vi "Emphasize Color.vi"(2 "error in 2 (no error)":errorcluster, 3 "Color":i8, 4 "Image Dst":T1, 5 "Image Src":T1) -> (0 "error out":errorcluster, 1 "Image Out":T1)   [LabVIEW 2009, in "ImageProcessing.lvlib"]
doc: "Output is a grayscaled image calculated as\n (255*X)/(R+G+B) \nwhere X is R, G or B depending on what number is showsen in color (0 = R, 1 = G, 2 = B)."
uses:
  <vilib>/vision/Image Controls.llb/IMAQ Image.ctl
  <vilib>/Analysis/Matrix/Numeric/Conversions/Matrix To Array - RM.vi
  <vilib>/Analysis/Matrix/Numeric/Add/Add - RM,RM.vi
  <vilib>/Analysis/Matrix/Numeric/Multiply/Multiply - RM,R.vi
  <vilib>/Analysis/Matrix/Numeric/Conversions/Array To Matrix - RA2.vi
  ImageProcessing.lvlib
  <vilib>/vision/NI_Vision_Development_Module.lvlib
  <vilib>/Analysis/Matrix/NI_Matrix.lvlib
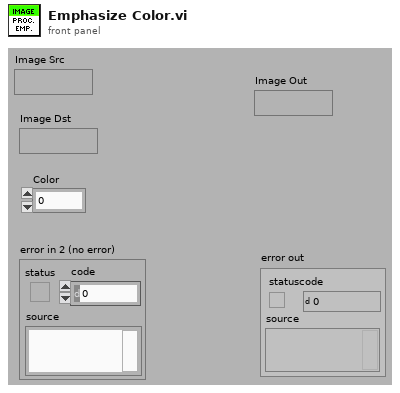
[diagram p1: front panel]
types:
  T1 = typedef "IMAQ Image.ctl" = refnum<image>
  T2 = typedef "NI_Matrix.lvlib/RealMatrix.ctl" = dbl[][]
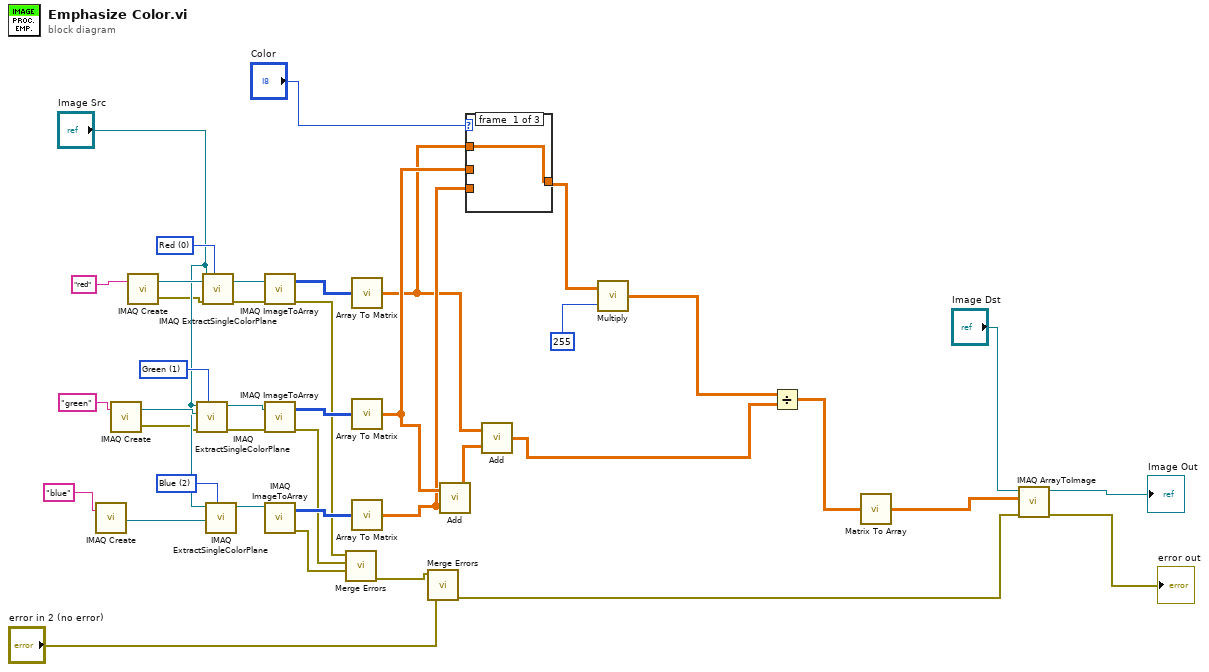
[diagram p0: block diagram]
diagram:
  w32 = 2 items=["Red", "Green", "Blue", "Hue", "Saturation", "Luminance", "Value", "Intensity"] ("Color Plane")
  w33 = 1 items=["Red", "Green", "Blue", "Hue", "Saturation", "Luminance", "Value", "Intensity"] ("Color Plane")
  w34 = 0 items=["Red", "Green", "Blue", "Hue", "Saturation", "Luminance", "Value", "Intensity"] ("Color Plane")
  n1 = call "IMAQ Create"("Image Name"="blue") -> ("New Image"=w35:T1)  [unwired: 3 in, 2 out]
  n2 = call "IMAQ Create"("Image Name"="green") -> ("New Image"=w36:T1, "error out"=w8:errorcluster)  [unwired: 3 in, 1 out]
  n3 = call "IMAQ Create"("Image Name"="red") -> ("New Image"=w37:T1, "error out"=w10:errorcluster)  [unwired: 3 in, 1 out]
  n4 = call "IMAQ ExtractSingleColorPlane"("Color Plane"=w33, "error in (no error)"=w8, "Image Dst"=w36, "Image Src"="Image Src") -> ("error out"=w7:errorcluster, "Image Dst Out"=w29:T1)  [unwired: 6 in]
  n5 = call "IMAQ ExtractSingleColorPlane"("Color Plane"=w34, "error in (no error)"=w10, "Image Dst"=w37, "Image Src"="Image Src") -> ("error out"=w9:errorcluster, "Image Dst Out"=w31:T1)  [unwired: 6 in]
  n6 = call "IMAQ ExtractSingleColorPlane"("Color Plane"=w32, "Image Dst"=w35, "Image Src"="Image Src") -> ("Image Dst Out"=w30:T1)  [unwired: 7 in, 1 out]
  n7 = call "IMAQ ImageToArray"("error in (no error)"=w9, "Image"=w31) -> ("error out"=w6:errorcluster, "Image Pixels (U8)"=w28:u8[][])  [unwired: 2 in, 3 out]
  n8 = call "IMAQ ImageToArray"("error in (no error)"=w7, "Image"=w29) -> ("error out"=w5:errorcluster, "Image Pixels (U8)"=w27:u8[][])  [unwired: 2 in, 3 out]
  n9 = call "IMAQ ImageToArray"("Image"=w30) -> ("error out"=w4:errorcluster, "Image Pixels (U8)"=w26:u8[][])  [unwired: 3 in, 3 out]
  n10 = call <vilib>:"Merge Errors.vi"("error in 3 (no error)"=w4, "error in 2 (no error)"=w5, "error in 1 (no error)"=w6) -> ("error out"=w2:errorcluster)  [unwired: 4 in]
  n11 = call-poly <vilib>:"Array To Matrix.vi"("Real 2D Array"=w28) -> ("Real Matrix"=w13:T2)
  n12 = call-poly <vilib>:"Array To Matrix.vi"("Real 2D Array"=w27) -> ("Real Matrix"=w16:T2)
  n13 = call-poly <vilib>:"Array To Matrix.vi"("Real 2D Array"=w26) -> ("Real Matrix"=w15:T2)
  n14 = call <vilib>:"Merge Errors.vi"("error in 2 (no error)"="error in 2 (no error)", "error in 1 (no error)"=w2) -> ("error out"=w3:errorcluster)  [unwired: 5 in]
  n15 = call-poly <vilib>:"Add.vi"("Real Matrix B"=w15, "Real Matrix A"=w16) -> ("A + B"=w25:T2)
  n16 = case shown="..0" "Color" {
    tunnel: w13 -> [w41 _ _]
    tunnel: w16 -> [_ w42 _]
    tunnel: w15 -> [_ _ w43]
    tunnel: [w41 w42 w43] -> w12
    frame #0 {
    }
    frame #1 {
    }
    frame #2 {
    }
  }
  n17 = call-poly <vilib>:"Add.vi"("Real Matrix B"=w25, "Real Matrix A"=w13) -> ("A + B"=w23:T2)
  n18 = call-poly <vilib>:"Multiply.vi"("Real Scalar c"=255, "Real Matrix A"=w12) -> ("A * c"=w22:T2)
  n19 = Divide(x=w22, y=w23) -> (x/y=w21:T2)
  n20 = call-poly <vilib>:"Matrix To Array.vi"("Real Matrix"=w21) -> ("Real 2D Array"=w20:dbl[][])
  n21 = call "IMAQ ArrayToImage"("error in (no error)"=w3, "Image Pixels (U8)"=w20, "Image"="Image Dst") -> ("error out"=→"error out":errorcluster, "Image Out"=→"Image Out":T1)  [unwired: 7 in]
